vi "Insert buffer element.vi"(8 "error in (no error)":errorcluster, 9 "DM":string, 10 "Serial":string, 11 "Domino Laser module Class in":refnum<class "Domino Laser module Class.lvclass">) -> (0 "error out":errorcluster, 2 "element inserted successfully":bool, 3 "Domino Laser module Class out":refnum<class "Domino Laser module Class.lvclass">)   [LabVIEW 2015, in "Domino LM.lvlib" / "Domino Laser module Class.lvclass"]
uses:
  CTRLS/Domino Laser module Class.lvclass
  Domino LM.lvlib
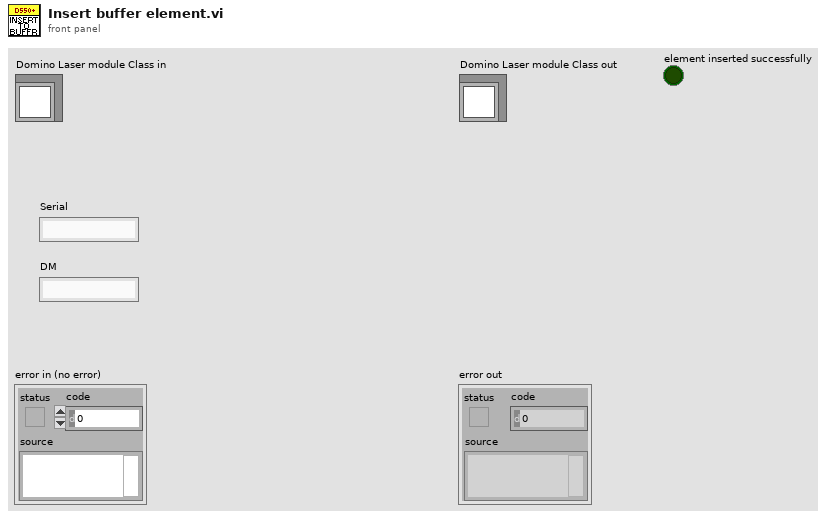
[diagram p1: front panel]
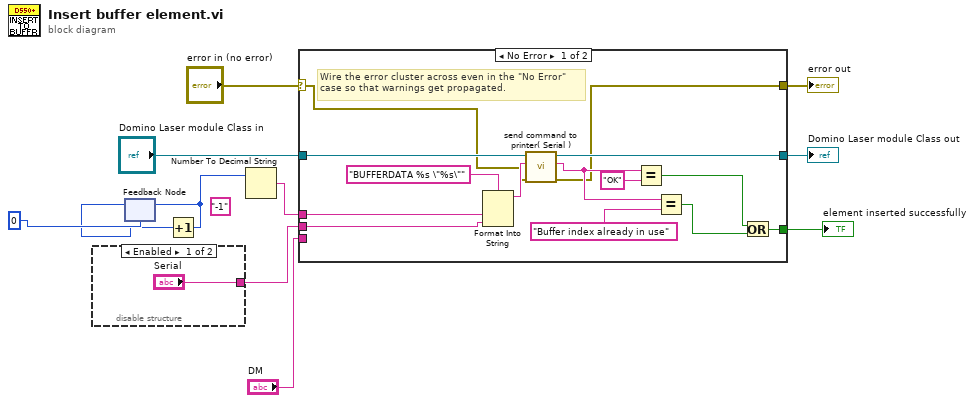
[diagram p0: block diagram]
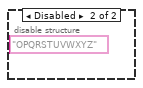
[diagram p2: hidden frame]
diagram:
  (unwired) "-1" ("buffer ID")
  n1 = disable-structure shown="Enabled" {
    disable-tunnel: ["Serial" _] -> w7
    frame Enabled {
    }
    frame Disabled {
      (unwired) "OPQRSTUVWXYZ" ("Text")
    }
  }
  n2 = feedback #1(u32 0) -> (w3:u32)
  n3 = Increment(x=w3) -> (x+1=w2:u32)
  n4 = feedback-in #1(w2) -> ()
  n5 = Number To Decimal String(number=w2) -> (decimal integer string=w1:string)  [unwired: 1 in]
  n6 = case shown="No Error" "error in (no error)" {
    selector: "error in (no error)" -> [w14 w28]
    tunnel: [w13 w28] -> w10
    tunnel: [w22 w27] -> w8
    tunnel: "Domino Laser module Class in" -> [w23 w27]
    tunnel: w1 -> [w25 _]
    tunnel: w7 -> [w24 _]
    tunnel: "DM" -> [_ _]
    tunnel: [w17 _] -> w5
    frame No Error {
      # "Wire the error cluster across even in the \"No Error\"\ncase so that warnings get propagated."
      n7 = Format Into String(format string="BUFFERDATA %s \"%s\"", w25, w24) -> (resulting string=w21:string)  [unwired: 2 in, 1 out]
      n8 = call "send command to printer( Serial ).vi"("error in (no error)"=w14, "command to be sent"=w21, "Domino Laser module Class in"=w23) -> ("error out"=w13:errorcluster, "Recived message"=w19:string, "Domino Laser module Class out"=w22:refnum<class "Domino Laser module Class.lvclass">)  [unwired: 5 in, 1 out]
      n9 = Equal?(x=w19, y="OK") -> (x = y?=w16:bool)
      n10 = Equal?(x=w19, y="Buffer index already in use" ("format string")) -> (x = y?=w15:bool)
      n11 = Or(x=w16, y=w15) -> (x .or. y?=w17:bool)
    }
    frame Error {
    }
  }
  "error out" <- w10
  "Domino Laser module Class out" <- w8
  "element inserted successfully" <- w5
